vi "LookupID.Create.vi"(9 "Serivce ID":u32, 10 "Service Type":T1, 11 "Direction":T2(ring)) -> (3 "Result":u64)   [LabVIEW 2019, in "Diagnostics Addon Shared.lvlib"]
uses:
  Diagnostics Addon Shared.lvlib
  Types/Type.ctl
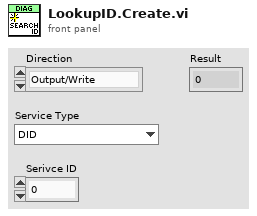
[diagram p1: front panel]
types:
  T1 = typedef "Diagnostics Addon Shared.lvlib/Type.ctl" = enum16{"DID", "CDID", "PID", "CPID", "Read Memory", "Write Memory", "IO Control", "Routine Start", "Routine Request", "Routine Stop", "User Defined", "DTC Control", "Clear DTCs", "Read DTCs", "Start DTCs", "DTC Change Count", "Tester Present", "Unlock ECU", "Reset ECU", "Diag Session Control", "Communication Control", "DPID Control", "Poll Control", "Diag CAN Control"}
  T2 = enum16{"Output/Write", "Input/Read", "Input/ReadWrite"}
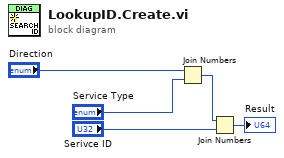
[diagram p0: block diagram]
diagram:
  n1 = Join Numbers(hi="Direction", lo="Service Type") -> ((hi.lo)=w4:u32)
  n2 = Join Numbers(hi=w4, lo="Serivce ID") -> ((hi.lo)=→"Result":u64)
